vi "linearFitCalc.vi"(8 "ready for output (T)":bool=TRUE, 9 "inputValid":bool=TRUE, 11 "input":T1) -> (0 "ready for input":bool, 1 "outputValid":bool=TRUE, 3 "output":cluster{"slope":fxp<+/-,22,1>, "forward":bool})   [LabVIEW 2016]
uses:
  <vilib>/rvi/Memory/Memory_Emulation/nirvimemoryFastEmulation.vi
  <vilib>/rvi/Memory/Memory_Emulation/nirvimemoryEmulation.vi
  <vilib>/rvi/Emulation/niFpgaEmulationIsFPGAContextNoSignature.vi
  <vilib>/rvi/DataTransferAndStorage/Container/Common/niFpgaContainerGetUniqueNameForEmu.vi
  <vilib>/rvi/Emulation/niFpgaProcessEmulError.vi
  <vilib>/rvi/Emulation/niFpgaSctlEmulationGetInTimedLoop.vi
  <vilib>/rvi/errors/nirviReportUnexpectedCaseInternalError (U32).vi
  <vilib>/rvi/FXPMathLib/FxpInterpret/XNode/nifxpmath_Interpret.xnode
  <vilib>/rvi/FXPMathLib/FxpMul/XNode/nifxpmath_Multiplier.xnode
  <vilib>/rvi/DataTransferAndStorage/Container/XNode/niFpgaContainer.xnode
  <vilib>/rvi/FXPMathLib/FxpAdd/XNode/nifxpmath_Add.xnode
  <vilib>/rvi/FXPMathLib/sim/FxpSim.dll
panel:
  out "fitParamsBwd":T2
  out "aCoeff":fxp<+/-,53,39>
  out "bCoeff":fxp<+/-,64,41>
  out "slope":fxp<+/-,22,20>
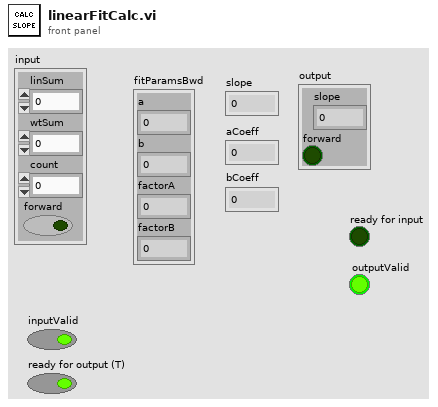
[diagram p1: front panel]
types:
  T1 = cluster{"linSum":i32, "wtSum":fxp<+/-,54,34>, "count":u16, "forward":bool}
  T2 = cluster{"a":fxp<+/-,21,7>, "b":fxp<+/-,21,7>, "factorA":i8, "factorB":i8}
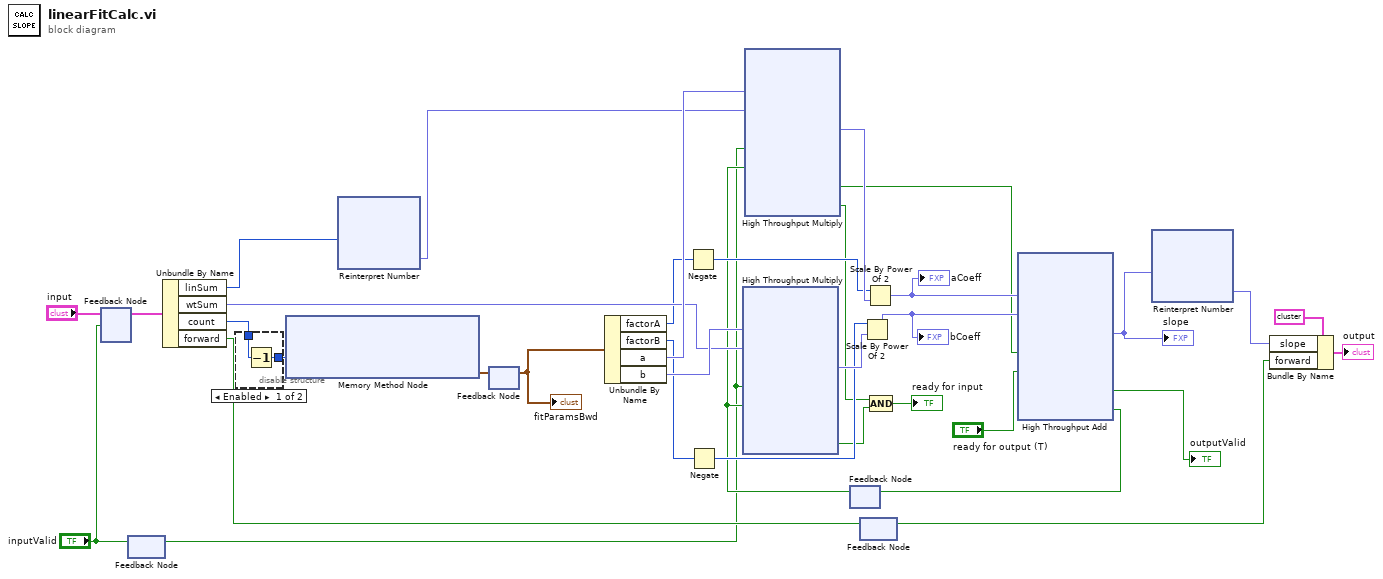
[diagram p0: block diagram]
diagram:
  n1 = feedback-in #1("input", "inputValid") -> ()
  n2 = feedback #1() -> (w4:T1)  [unwired: 1 in]
  n3 = feedback-in #2("inputValid") -> ()
  n4 = feedback #2() -> (w5:bool)  [unwired: 1 in]
  n5 = Unbundle By Name(w4) -> ("linSum"=w30:i32, "wtSum"=w31:fxp<+/-,54,34>, "count"=w35:u16, "forward"=w17:bool)
  n6 = disable-structure shown="Enabled" {
    disable-tunnel: w35 -> [w37 w38]
    disable-tunnel: [w36 w38] -> w1
    frame Enabled {
      n7 = Decrement(x=w37) -> (x-1=w36:u16)
    }
    frame Disabled {
    }
  }
  n8 = xnode ("Memory Method Node")("Address"=w1) -> ("Data"=w34:T2)  [unwired: 1 in, 1 out]
  n9 = xnode "Reinterpret Number"("x"=w30) -> ("y"=w29:fxp<+/-,32,32>)
  n10 = feedback-in #3(w34) -> ()
  n11 = feedback #3() -> (w7:T2)  [unwired: 1 in]
  "fitParamsBwd" <- w7
  n12 = Unbundle By Name(w7) -> ("factorA"=w24:i8, "factorB"=w23:i8, "a"=w33:fxp<+/-,21,7>, "b"=w32:fxp<+/-,21,7>)
  n13 = Negate(x=w24) -> (-x=w22:i8)
  n14 = Negate(x=w23) -> (-x=w21:i8)
  n15 = feedback #4() -> (w9:bool)  [unwired: 1 in]
  n16 = xnode ("High Throughput Multiply")("x"=w32, "y"=w31, "input valid"=w5, "ready for output (T)"=w9) -> ("x*y"=w28:fxp<+/-,64,41>, "ready for input"=w15:bool)  [unwired: 1 out]
  n17 = xnode ("High Throughput Multiply")("x"=w33, "y"=w29, "input valid"=w5, "ready for output (T)"=w9) -> ("x*y"=w27:fxp<+/-,53,39>, "output valid"=w11:bool, "ready for input"=w16:bool)
  n18 = feedback-in #5(w17) -> ()
  n19 = feedback #5() -> (w2:bool)  [unwired: 1 in]
  n20 = Scale By Power Of 2(n=w21, x=w28) -> (x*2^n=w25:fxp<+/-,64,41>)
  "bCoeff" <- w25
  n21 = Scale By Power Of 2(n=w22, x=w27) -> (x*2^n=w26:fxp<+/-,53,39>)
  "aCoeff" <- w26
  n22 = Compound Arithmetic op=AND(w16, w15) -> (→"ready for input":bool)
  n23 = xnode ("High Throughput Add")("x"=w26, "y"=w25, "input valid"=w11, "ready for output (T)"="ready for output (T)") -> ("x+y"=w18:fxp<+/-,22,20>, "output valid"=→"outputValid":bool, "ready for input"=w10:bool)
  "slope" <- w18
  n24 = feedback-in #4(w10) -> ()
  n25 = xnode "Reinterpret Number"("x"=w18) -> ("y"=w13:fxp<+/-,22,1>)
  n26 = Bundle By Name(cluster=cluster{"slope":fxp<+/-,22,1>, "forward":bool} {"slope"=0.0, "forward"=FALSE} ("Cluster"), "slope"=w13, "forward"=w2) -> (→"output":cluster{"slope":fxp<+/-,22,1>, "forward":bool})
